vi "LoginUser.vi"(8 "error in (no error)":errorcluster, 9 "LastUserName":string, 10 "IsInitialLogin":bool, 11 "Sequence Context In":refnum<k7>) -> (0 "error out":errorcluster, 3 "logOut":bool)   [LabVIEW 2019]
doc: "This is the top level VI called by the FrontEndCallbacks.seq file to launch and manage the login process in TestStand. To use this VI instead of the default CVI code to manage the login dialog, open the FrontEndCallbacks sequence (<TestStand Public>\\Components\\Callbacks\\Station\\StationCallbacks.seq), set the first two steps to \"skip\" and the last two to normal in run mode. Note: this code differs from the CVI version in that The users are selected by a ring control, and must be chosen; names cannot be manually typed"
panel:
  out "Sequence Context Out":refnum<k7>
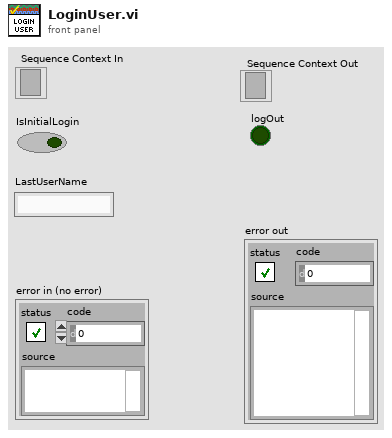
[diagram p1: front panel]
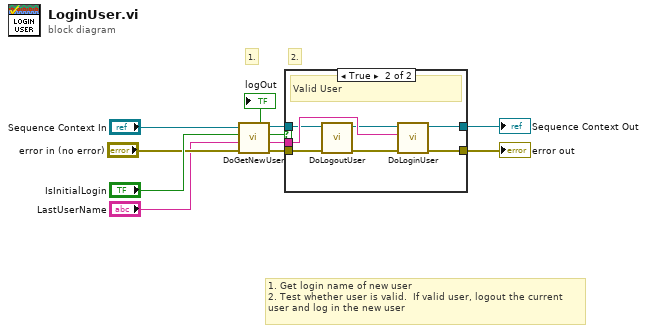
[diagram p0: block diagram]
diagram:
  # "1. Get login name of new user\n2. Test whether user is valid.  If valid user, logout the current user and log in the new user"
  # "1."
  # "2."
  n1 = call "DoGetNewUser.vi"("error in (no error)"="error in (no error)", "LastUserName"="LastUserName", "IsInitialLogin"="IsInitialLogin", "Sequence Context In"="Sequence Context In") -> ("error out"=w8:errorcluster, "LoginName"=w6:string, "isValidUser"=w9:bool, "Sequence Context Out"=w3:refnum<k7>, "logOut"=→"logOut":bool)  [unwired: 3 in]
  n2 = case shown="True" w9 {
    tunnel: w3 -> [w13 w16]
    tunnel: w8 -> [w12 w20]
    tunnel: [w13 w19] -> w5
    tunnel: [w12 w18] -> w2
    tunnel: w6 -> [_ w17]
    frame False {
      # "Invalid User"
    }
    frame True {
      # "Valid User"
      n3 = call "DoLogoutUser.vi"("error in (no error)"=w20, "Sequence Context In"=w16) -> ("error out"=w15:errorcluster, "Sequence Context Out"=w14:refnum<k7>)  [unwired: 6 in]
      n4 = call "DoLoginUser.vi"("error in (no error)"=w15, "LoginName"=w17, "Sequence Context In"=w14) -> ("error out"=w18:errorcluster, "Sequence Context Out"=w19:refnum<k7>)  [unwired: 5 in]
    }
  }
  "error out" <- w2
  "Sequence Context Out" <- w5
